vi "Pre Launch Init.vi"(11 "LED Matrix in":refnum<class "LED Matrix.lvclass">) -> (0 "error out":errorcluster, 3 "LED Matrix out":refnum<class "LED Matrix.lvclass">)   [LabVIEW 2026, in "LED Matrix.lvlib" / "LED Matrix.lvclass"]
doc: "<p>(<strong>Filename</strong>: <span class=\"dnl\">Actor Framework.lvlib:Actor.lvclass:Pre Launch Init.vi</span>)</p>\n<p>Defines behavior that occurs after the <a href=\"nihelplauncher://docs/csh?context=lvcore_lvcomm_af_launch_nested_actor\">Launch Nested Actor</a> method is invoked but before the actor's Actor Core method begins running.</p>\n<p>By default, this method does nothing. A descendant class may override it to define behavior.</p>"
uses:
  LED Matrix.lvclass
  LED Matrix.lvclass/LED Matrix.ctl
  <vilib>/ActorFramework/Actor/Actor.lvclass
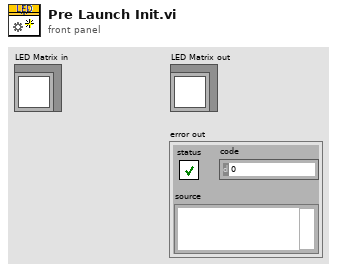
[diagram p1: front panel]
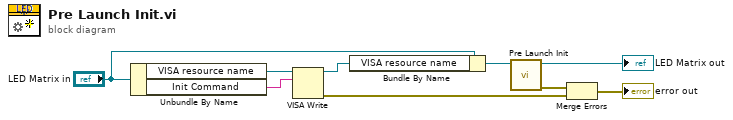
[diagram p0: block diagram]
diagram:
  n1 = Unbundle By Name("LED Matrix in") -> ("VISA resource name"=w6:refnum<visa-resource-name>, "Init Command"=w3:string)
  n2 = VISA Write(VISA resource name=w6, write buffer=w3) -> (VISA resource name out=w4:refnum<visa-resource-name>, error out=w1:errorcluster)  [unwired: 1 in, 1 out]
  n3 = Bundle By Name(cluster="LED Matrix in", "VISA resource name"=w4) -> (w5:refnum<class "LED Matrix.lvclass">)
  n4 = call-parent "Pre Launch Init.vi"("Actor in"=w5) -> ("error out"=w9:errorcluster, "Actor out"=→"LED Matrix out":refnum<class "LED Matrix.lvclass">)  [unwired: 9 in]
  n5 = Merge Errors(w9, w1) -> (→"error out":errorcluster)
